vi "Load Index.vi"(8 "error in (no error)":errorcluster, 10 "Project Path":path) -> (0 "error out":errorcluster, 3 "Test Finder out":refnum<class "Test Finder.lvclass">)   [LabVIEW 2020, in "Test Finder.lvclass"]
uses:
  Test Finder.lvclass
  LUnit Test Suite.lvclass
  Index.ctl
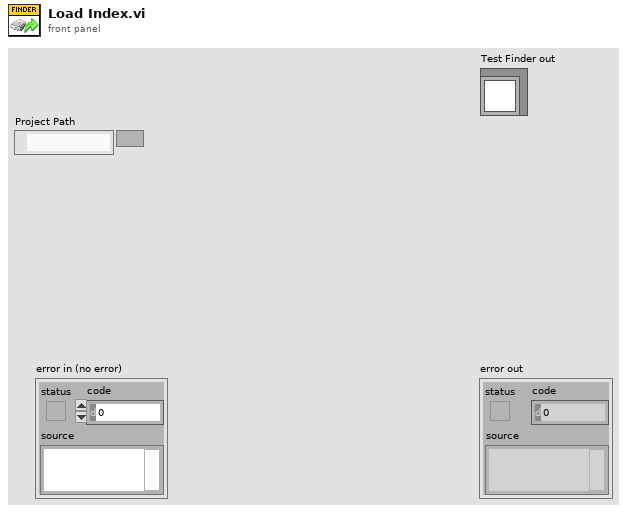
[diagram p1: front panel]
types:
  T1 = enum16{"open", "replace", "create", "open or create", "replace or create", "replace or create with confirmation"}
  T2 = typedef "Test Finder.lvclass/Index.ctl" = cluster{"Checksums":map{path, string}, "Suite":refnum<class "LUnit Test Suite.lvclass">}
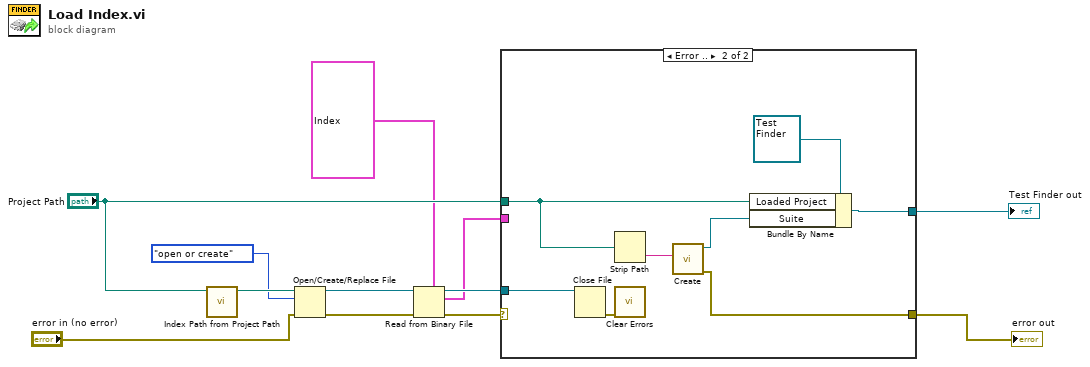
[diagram p0: block diagram]
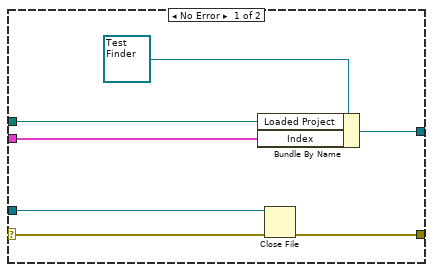
[diagram p2: hidden frame]
diagram:
  n1 = call "Index Path from Project Path.vi"("Project Path"="Project Path") -> ("appended path"=w9:path)  [unwired: 10 in]
  n2 = Open/Create/Replace File(file path (use dialog)=w9, error in="error in (no error)", operation (0:open)=T1."open or create") -> (refnum out=w8:refnum<file>, error out=w2:errorcluster)  [unwired: 3 in, 1 out]
  n3 = Read from Binary File(5:T2 {"Checksums"={}, "Suite"=refnum} ("Index"), 8:w2, 11:w8) -> (0:w1:errorcluster, 2:w5:T2, 3:w6:refnum<file>)  [unwired: 3 in, 1 out]
  n4 = case shown="Error .." w1 {
    selector: w1 -> [w13 _]
    tunnel: [w18 w26] -> w12
    tunnel: "Project Path" -> [w17 w24]
    tunnel: [w16 w21] -> w7
    tunnel: w6 -> [w15 w25]
    tunnel: w5 -> [w14 _]
    frame No Error {
      n5 = Bundle By Name(cluster=refnum<class "Test Finder.lvclass"> refnum ("Test Finder in"), "Loaded Project"=w17, "Index"=w14) -> (w18:refnum<class "Test Finder.lvclass">)
      n6 = Close File(refnum=w15, error in=w13) -> (error out=w16:errorcluster)  [unwired: 1 out]
    }
    frame Error {
      n7 = Close File(refnum=w25) -> (error out=w20:errorcluster)  [unwired: 1 in, 1 out]
      n8 = Strip Path(path=w24) -> (name=w23:string)  [unwired: 1 out]
      n9 = call <vilib>:"Clear Errors.vi"("error in (no error)"=w20) -> ()  [unwired: 5 in, 2 out]
      n10 = call "Create.vi"("Suite Name"=w23) -> ("error out"=w21:errorcluster, "LUnit Test Suite Out"=w22:refnum<class "LUnit Test Suite.lvclass">)  [unwired: 9 in]
      n11 = Bundle By Name(cluster=refnum<class "Test Finder.lvclass"> refnum ("Test Finder in"), "Loaded Project"=w24, "Suite"=w22) -> (w26:refnum<class "Test Finder.lvclass">)
    }
  }
  "error out" <- w7
  "Test Finder out" <- w12
